vi "send_elemszam.vi"() -> ()   [LabVIEW 2013]
panel:
  in  "elemszam":u16
  out "error out":errorcluster
  out "VISA resource name out":refnum<visa-resource-name>
  in  "VISA resource name 3":refnum<visa-resource-name>
  in  "error in (no error) 3":errorcluster
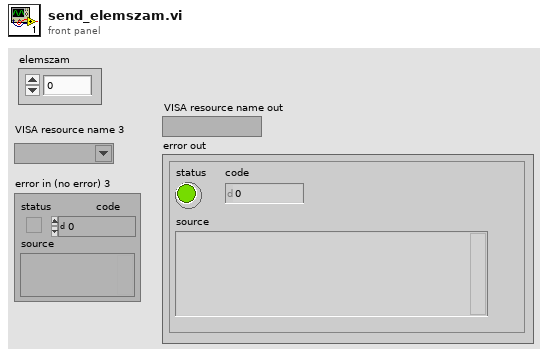
[diagram p1: front panel]
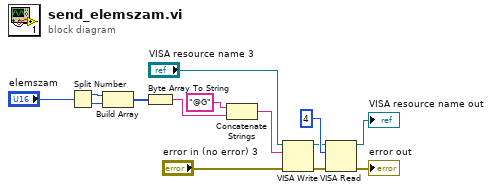
[diagram p0: block diagram]
diagram:
  n1 = Split Number(x="elemszam") -> (hi(x)=w4:u8, lo(x)=w3:u8)
  n2 = Build Array(w4, w3) -> (w2:u8[])
  n3 = Byte Array To String(unsigned byte array=w2) -> (string=w1:string)
  n4 = Concatenate Strings("@G" ("write buffer"), w1) -> (w11:string)
  n5 = VISA Write(VISA resource name="VISA resource name 3", write buffer=w11, error in (no error)="error in (no error) 3") -> (VISA resource name out=w9:refnum<visa-resource-name>, error out=w8:errorcluster)  [unwired: 1 out]
  n6 = VISA Read(VISA resource name=w9, byte count=u32 4, error in (no error)=w8) -> (VISA resource name out=→"VISA resource name out":refnum<visa-resource-name>, error out=→"error out":errorcluster)  [unwired: 2 out]
